vi "PH_Meter.vi"() -> ()   [LabVIEW 2018]
uses:
  <vilib>/Instr/_visa.llb/VISA Configure Serial Port (Instr).vi
panel:
  out "Waveform Chart":dbl(graph)=6.13
  out "PH":dbl=6.13
  out "number 3":i32=6
  out "substring 3":string="6"
  out "number 2":i32
  out "substring 2":string="0"
  in  "offset":i32=2
  out "number":i32=13
  out "substring":string="6.13"
  out "read buffer":string="P+06.13T+023.1M+0042\r\n"
  in  "stop":bool
  in  "VISA resource name 2":refnum<visa-resource-name>="COM3"
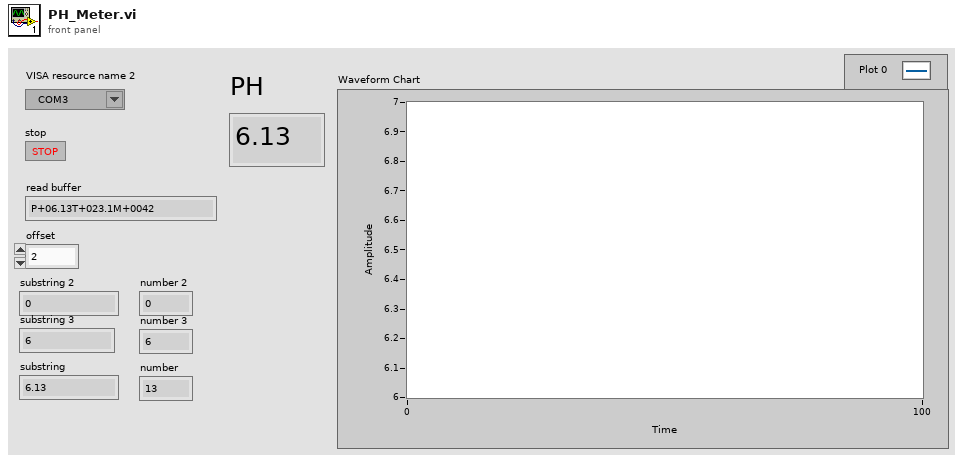
[diagram p1: front panel]
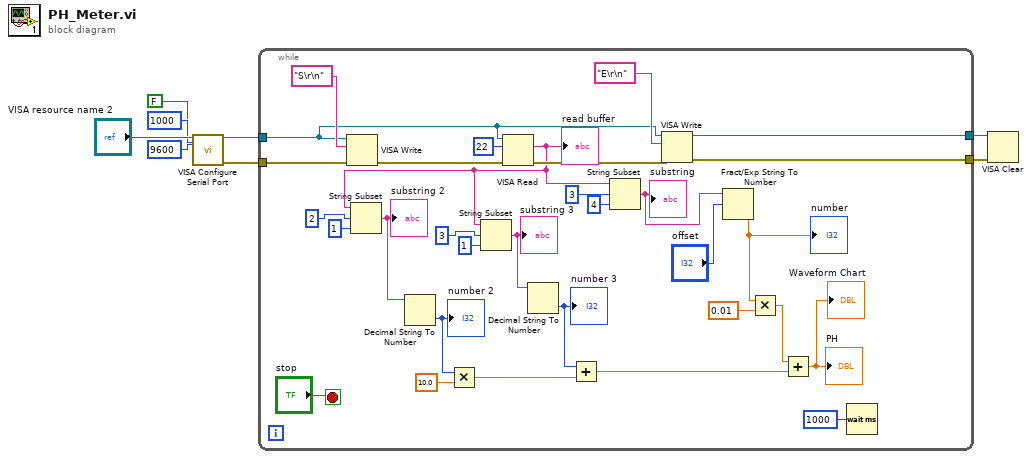
[diagram p0: block diagram]
diagram:
  n1 = call-poly "VISA Configure Serial Port"("VISA resource name"="VISA resource name 2", "timeout (10sec)"=u32 1000, "Enable Termination\nChar (T)"=FALSE ("Enable Termination\nChar (T)"), "baud rate (9600)"=u32 9600) -> ("VISA resource name out"=w8:refnum<visa-resource-name>, "error out"=w3:errorcluster)  [unwired: 10 in]
  n2 = while {
    tunnel: w8 -> [w28]
    tunnel: w3 -> [w38]
    tunnel: [w27] -> w2
    tunnel: [w26] -> w1
    stop <- "stop" stop-if-true
    n3 = VISA Write(VISA resource name=w28, write buffer="S\r\n" ("string"), error in (no error)=w38) -> (error out=w39:errorcluster)  [unwired: 2 out]
    n4 = VISA Read(VISA resource name=w28, byte count=u32 22, error in (no error)=w39) -> (read buffer=w19:string, error out=w34:errorcluster)  [unwired: 2 out]
    "read buffer" <- w19
    n5 = String Subset(string=w19, offset (0)=2, length (rest)=1 ("length (rest)")) -> (substring=w22:string)
    "substring 2" <- w22
    n6 = Decimal String To Number(string=w22) -> (number=w16:i32)  [unwired: 2 in, 1 out]
    "number 2" <- w16
    n7 = Multiply(x=w16, y=10.0) -> (x*y=w13:dbl)
    n8 = String Subset(string=w19, offset (0)=3, length (rest)=1 ("length (rest)")) -> (substring=w18:string)
    "substring 3" <- w18
    n9 = Decimal String To Number(string=w18) -> (number=w12:i32)  [unwired: 2 in, 1 out]
    "number 3" <- w12
    n10 = Add(x=w12, y=w13) -> (x+y=w11:dbl)
    n11 = String Subset(string=w19, offset (0)=3, length (rest)=4 ("length (rest)")) -> (substring=w29:string)
    "substring" <- w29
    n12 = VISA Write(VISA resource name=w28, write buffer="E\r\n" ("string"), error in (no error)=w34) -> (VISA resource name out=w27:refnum<visa-resource-name>, error out=w26:errorcluster)  [unwired: 1 out]
    n13 = Fract/Exp String To Number(string=w29, offset="offset") -> (number=w14:dbl)  [unwired: 2 in, 1 out]
    "number" <- w14
    n14 = Multiply(x=w14, y=0.01) -> (x*y=w10:dbl)
    n15 = Add(x=w10, y=w11) -> (x+y=→"PH" →"Waveform Chart":dbl)
    n16 = Wait (ms)(milliseconds to wait=u32 1000) -> ()  [unwired: 1 out]
  }
  n17 = VISA Clear(VISA resource name=w2, error in (no error)=w1) -> ()  [unwired: 2 out]
